vi "SubVI Tester.vi"() -> ()   [LabVIEW 2012]
panel:
  out "气象数据":T1={"当前温度"=29.937499999999993, "最高温度"=30.0, "最低温度"=10.0, "警告？"=FALSE, "警告文本"="无警告"}
  in  "最低温度":dbl=10.0
  in  "最高温度":dbl=30.0
  in  "停止":bool
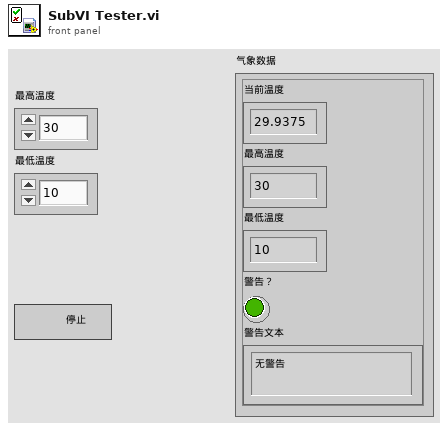
[diagram p1: front panel]
types:
  T1 = cluster{"当前温度":dbl, "最高温度":dbl, "最低温度":dbl, "警告？":bool, "警告文本":string}
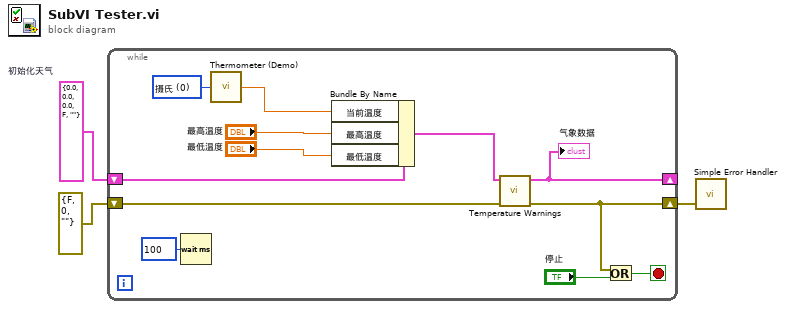
[diagram p0: block diagram]
diagram:
  w3 = T1 {"当前温度"=0.0, "最高温度"=0.0, "最低温度"=0.0, "警告？"=FALSE, "警告文本"=""}  # 初始化天气
  n1 = while {
    shift-right: [w10] -> _
    shift-left: w3 -> [w5]
    shift-right: [w11] -> w2
    shift-left: cluster{"状态":bool, "代码":i32, "源":string} {"状态"=FALSE, "代码"=0, "源"=""} ("错误输出") -> [w12]
    stop <- w13 stop-if-true
    w4 = u16 0 items=["摄氏", "华氏"] ("单位（0：摄氏度）")
    n2 = Wait (ms) ("等待(ms)")(milliseconds to wait=u32 100 ("等待时间（毫秒）")) -> ()  [unwired: 1 out]
    n3 = call "Thermometer (Demo).vi"("单位（0：摄氏度）"=w4) -> ("温度值"=w7:dbl)
    n4 = Bundle By Name ("按名称捆绑")(cluster=w5, "当前温度"=w7, "最高温度"="最高温度", "最低温度"="最低温度") -> (w6:T1)
    n5 = call "Temperature Warnings.vi"("错误输入"=w12, "气象数据输入"=w6) -> ("错误输出"=w11:cluster{"状态":bool, "代码":i32, "源":string}, "气象数据输出"=w10:T1)  [unwired: 8 in]
    "气象数据" <- w10
    n6 = Or ("或")(x=w11, y="停止") -> (x .or. y?=w13:bool)
  }
  n7 = call <vilib>:"Simple Error Handler.vi"("error in (no error)"=w2) -> ()  [unwired: 4 in, 5 out]
